vi "image_processing.vi"(9 "Input\nparameters":T3={"Frame rate (ms)"=2000, "Worm Strain"="N2", "Time t"=0, "State"=enum."Image acquisition", "Acquisition time"=0.0, "Maximum # of images"=100000, "#TTL"=0, "time of third ttl "=100000, "Image subtraction value"=0, "Time of last TTL"=0, "# Rows"=2, "# Columns"=2, "number of adjecentTTL"=0, "Sleep Deprivation status"="", "Sleep Detection"=FALSE, "Time of first sleep detection"=0, "# Sleep detections"=0, "Time max # adjacent TTL"=0, "Image t-1"=[], "Image t"=[]} {"# Columns" items=["1"=1, "2"=2, "3"=3, "4"=4]; "# Rows" items=["1"=1, "2"=2, "3"=3, "4"=4]}) -> (1 "Output \nparameters":T2={"Frame rate (ms)"=2000, "Worm strain"="N2", "Time t"=0, "State"=enum."Image acquisition", "Time elapsed"=0.0, "Max_num_runs"=100000, "#TTL"=0, "Time of start TTL"=100000, "ImSub Value"=0, "Time of last TTL"=0, "Number of Columns"=2, "Number of Rows"=2, "# AdjacentTTL"=0, "Sleep deprivation status"="", "Sleep Detection"=FALSE, "# Sleep detections"=0, "Time of first sleep detection"=0, "Time max # adjacent TTL"=0, "Image t-1"=[], "Image t"=[]} {"Number of Rows" items=["1"=1, "2"=2, "3"=3, "4"=4]; "Number of Columns" items=["1"=1, "2"=2, "3"=3, "4"=4]})   [LabVIEW 2011]
uses:
  state.ctl
  Action Items.ctl
  Action-Init-Update-Get.ctl
panel:
  # "General settings"
  # "Select number of animals"
  # "Row"
  # "Column"
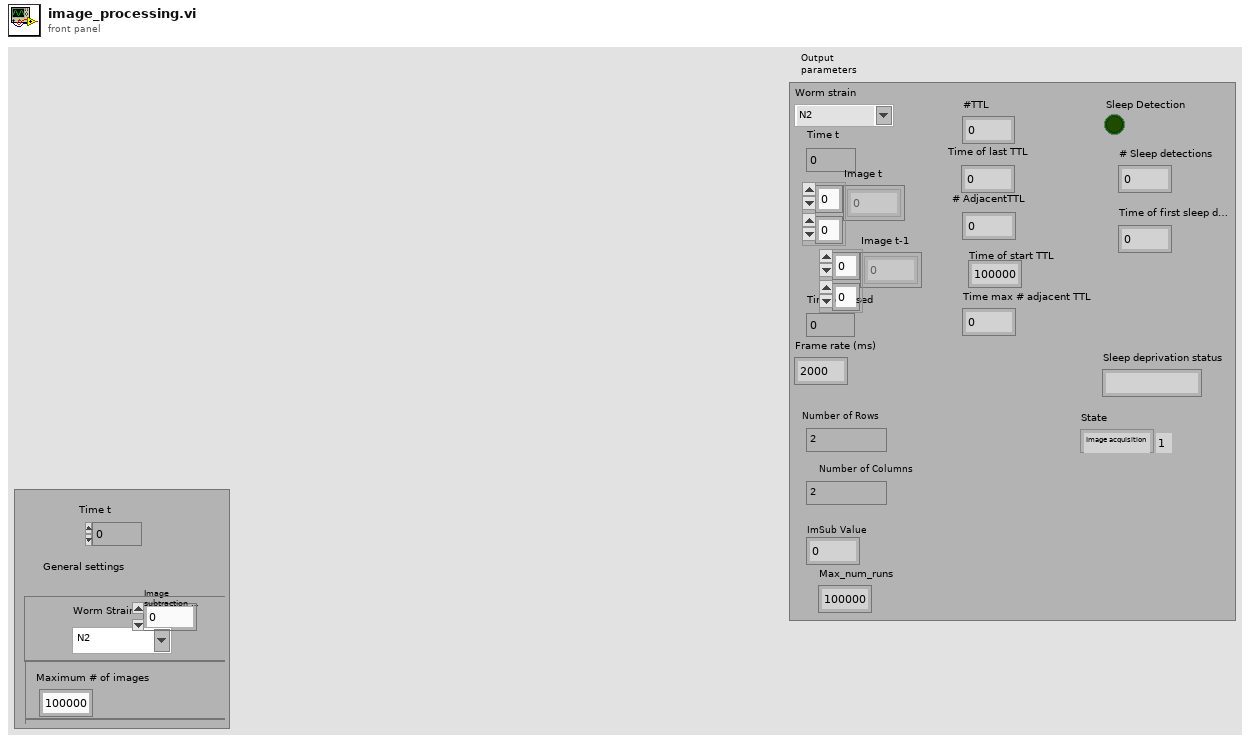
[diagram p1: front panel]
types:
  T1 = typedef "state.ctl" = enum16{"Initialize measurement", "Image acquisition", "Image processing", "Sleep detection", "Control TTL protocol ", "Sleep deprivation", "Update image & exit condition", "Wait "}
  T2 = cluster{"Frame rate (ms)":u32, "Worm strain":string, "Time t":i32, "State":T1, "Time elapsed":dbl, "Max_num_runs":i32, "#TTL":i32, "Time of start TTL":i32, "ImSub Value":i32, "Time of last TTL":i32, "Number of Columns":u32, "Number of Rows":u32, "# AdjacentTTL":i32, "Sleep deprivation status":string, "Sleep Detection":bool, "# Sleep detections":i32, "Time of first sleep detection":i32, "Time max # adjacent TTL":i32, "Image t-1":i32[][], "Image t":i32[][]}
  T3 = cluster{"Frame rate (ms)":u32, "Worm Strain":string, "Time t":i32, "State":T1, "Acquisition time":dbl, "Maximum # of images":i32, "#TTL":i32, "time of third ttl ":i32, "Image subtraction value":i32, "Time of last TTL":i32, "# Rows":u32, "# Columns":u32, "number of adjecentTTL":i32, "Sleep Deprivation status":string, "Sleep Detection":bool, "Time of first sleep detection":i32, "# Sleep detections":i32, "Time max # adjacent TTL":i32, "Image t-1":i32[][], "Image t":i32[][]}
  T4 = typedef "Action Items.ctl" = enum16{"Initialize", "Get"}
  T5 = typedef "Action-Init-Update-Get.ctl" = enum16{"Initialize", "Update", "Get"}
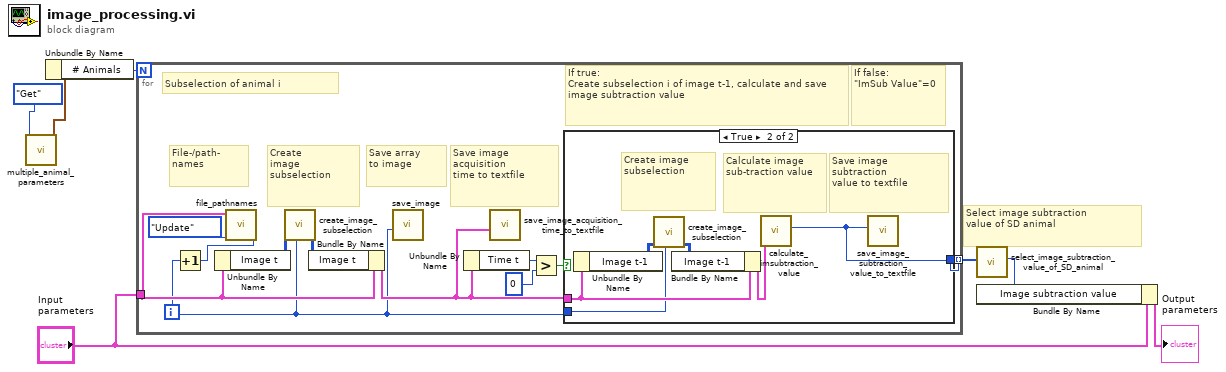
[diagram p0: block diagram]
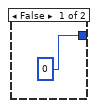
[diagram p2: hidden frame]
diagram:
  # "Select image subtraction\nvalue of SD animal"
  n1 = call "multiple_animal_parameters.vi"("Action"=Action_Items."Get") -> ("Animal\nparameters"=w6:cluster{"# Animals":i32, "Index SD animal":i32})  [unwired: 10 in]
  n2 = Unbundle By Name(w6) -> ("# Animals"=w5:i32)
  n3 = for {
    N: w5 -> [_]
    tunnel: "Input\nparameters" -> [w13]
    tunnel: [w12] -> w4 mode=indexing
    i -> [w9]
    # "Subselection of animal i"
    # "Save image\nacquisition\ntime to textfile"
    # "Save array\nto image"
    # "Create \nimage\nsubselection"
    # "If false:\n\"ImSub Value\"=0"
    # "If true: \nCreate subselection i of image t-1, calculate and save image subtraction value"
    # "File-/path-\nnames"
    n4 = Increment(x=w9) -> (x+1=w10:i32)
    n5 = Unbundle By Name(w13) -> ("Image t"=w18:i32[][])
    n6 = call "file_pathnames.vi"("Animal x"=w10, "Action"=Action-Init-Update-Get."Update", "Input \nparameters"=w13) -> ()  [unwired: 8 in, 1 out]
    n7 = call "create_image_subselection.vi"("Animal x"=w9, "Full image"=w18) -> ("Animal x\nimage subselection"=w17:i32[][])  [unwired: 9 in]
    n8 = Bundle By Name(cluster=w13, "Image t"=w17) -> (w11:T3)
    n9 = call "save_image.vi"("Image index"=w9) -> ()  [unwired: 11 in]
    n10 = Unbundle By Name(w11) -> ("Time t"=w16:i32)
    n11 = call "save_image_acquisition_time_to_textfile.vi"("Input \nparameters"=w11) -> ()  [unwired: 11 in]
    n12 = Greater?(x=w16, y=0) -> (0:w14:bool)
    n13 = case shown="True" w14 {
      tunnel: w11 -> [_ w23]
      tunnel: w9 -> [_ w22]
      tunnel: [0 ("ImSub Value") w21] -> w12
      frame False {
      }
      frame True {
        # "Save image\nsubtraction\nvalue to textfile"
        # "Create image subselection"
        # "Calculate image sub-traction value"
        n14 = Unbundle By Name(w23) -> ("Image t-1"=w25:i32[][])
        n15 = call "create_image_subselection.vi"("Animal x"=w22, "Full image"=w25) -> ("Animal x\nimage subselection"=w24:i32[][])  [unwired: 9 in]
        n16 = Bundle By Name(cluster=w23, "Image t-1"=w24) -> (w20:T3)
        n17 = call "calculate_imsubtraction_value.vi"("Input \nparameters"=w20) -> ("Image subtraction\nvalue"=w21:i32)  [unwired: 9 in, 1 out]
        n18 = call "save_image_subtraction_value_to_textfile.vi"("Image subtraction\nvalue"=w21) -> ()  [unwired: 11 in]
      }
    }
  }
  n19 = call "select_image_subtraction_value_of_SD_animal.vi"("Image subtraction \nvalues of all animals"=w4) -> ("Image subtraction \nvalue of SD animal"=w3:i32)  [unwired: 9 in]
  n20 = Bundle By Name(cluster="Input\nparameters", "Image subtraction value"=w3) -> (→"Output \nparameters":T3)
